vi "W5E2.vi"() -> ()   [LabVIEW 2021]
uses:
  <vilib>/LabVIEW Interface for Arduino/LabVIEW Interface for Arduino.lvlib
panel:
  out "x <= y?":bool
  out "Light Intensity (0 - 100)":dbl(knob) scale=0.0..100.0
  in  "Photo Cell Pin (0)":u8
  in  "VISA resource":refnum<visa-resource-name>
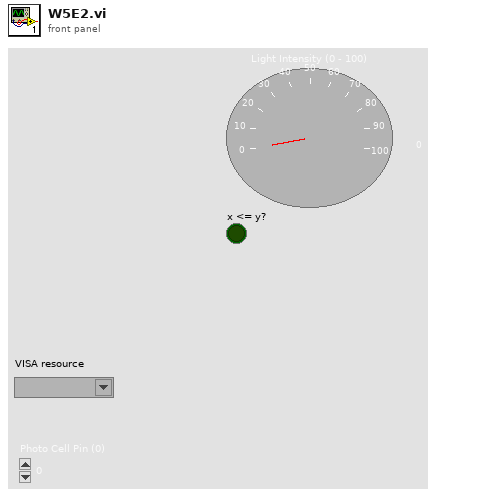
[diagram p1: front panel]
types:
  T1 = typedef "LabVIEW Interface for Arduino.lvlib/Arduino Resource.ctl" = cluster{"VISA resource":refnum<visa-resource-name>, "Board Type":T2, "Connection Type":enum8{"USB / Serial"}, "Bytes Per Packet (15)":u8}
  T2 = typedef "LabVIEW Interface for Arduino.lvlib/Board Type.ctl" = enum16{"Uno", "Dimuelanove w/Atmega 328", "Mega 2560"}
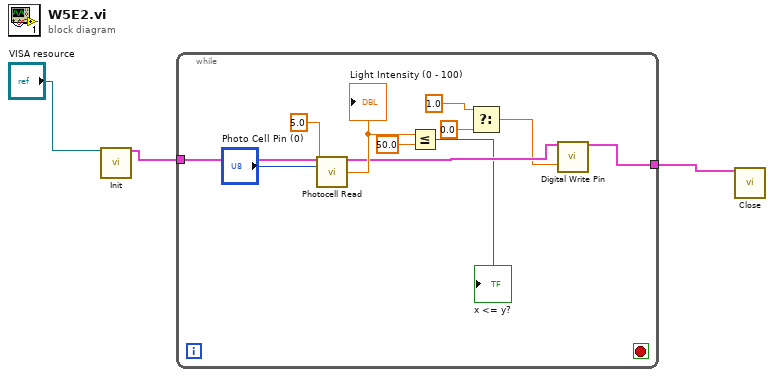
[diagram p0: block diagram]
diagram:
  n1 = call <vilib>:"Init.vi"("VISA resource"="VISA resource") -> ("Arduino Resource"=w2:T1)  [unwired: 17 in, 1 out]
  n2 = while {
    tunnel: w2 -> [w14]
    tunnel: [w6] -> w1
    stop <- _ stop-if-true
    n3 = call <vilib>:"Photocell Read.vi"("Arduino Resource"=w14, "Photo Cell Pin (0)"="Photo Cell Pin (0)", "Vcc (5)"=5.0) -> ("Arduino Resource"=w7:T1, "Light Intensity (0 - 100)"=w11:dbl)  [unwired: 10 in, 1 out]
    "Light Intensity (0 - 100)" <- w11
    n4 = Less Or Equal?(x=w11, y=50.0) -> (x <= y?=→"x <= y?":bool)
    n5 = Select(t=1.0, f=0.0) -> (s? t:f=w5:dbl)  [unwired: 1 in]
    n6 = call <vilib>:"Digital Write Pin.vi"("Arduino Resource"=w7, "Value (0)"=w5) -> ("Arduino Resource"=w6:T1)  [unwired: 12 in, 1 out]
  }
  n7 = call <vilib>:"Close.vi"("Arduino Resource"=w1) -> ()  [unwired: 14 in, 1 out]
